vi "Fetch.vi"   [LabVIEW 2021, in "Keithley 24XX.lvlib"]
doc: "Fetches acquired data from the instrument. The correct fetch subVI depends on the desired data."
uses:
  <instrlib>/Keithley 24XX/Keithley 24XX.lvlib
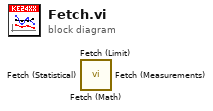
[diagram p0: block diagram]
diagram:
  n1 = call <instrlib>:"Fetch (Math).vi"() -> ()  [unwired: 13 in, 3 out]
  n2 = call <instrlib>:"Fetch (Limit).vi"() -> ()  [unwired: 13 in, 3 out]
  n3 = call <instrlib>:"Fetch (Statistical).vi"() -> ()  [unwired: 13 in, 3 out]
  n4 = call <instrlib>:"Fetch (Measurements).vi"() -> ()  [unwired: 9 in, 7 out]
